vi "Populate Method Results.vi"(8 "error in (no error)":errorcluster, 10 "Test Method Result":refnum<class "Method Result.lvclass">, 11 "Test Tree In":refnum<class "Test Result Tree.lvclass">) -> (0 "error out":errorcluster, 2 "Test Method Result Out":refnum<class "Method Result.lvclass">, 3 "Test Tree Out":refnum<class "Test Result Tree.lvclass">)   [LabVIEW 2020, in "Test Result Tree.lvclass"]
uses:
  Test Result Tree/Test Result Tree.lvclass
  C:/Users/anton/Documents/GitHub/LUnit/source/Framework/Helper Classes/Test Tree/Test Tree.lvclass
  Result Classes/Method Result/Method Result.lvclass
  Test Tree.lvclass/Test Tree.ctl
  Result Classes/Method Result/Method Result.lvclass/Method Result.ctl
  Test Tree.lvclass
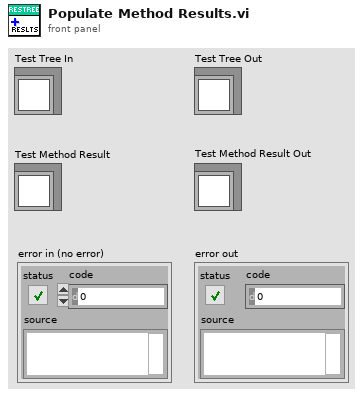
[diagram p1: front panel]
types:
  T1 = map{string, cluster{"Left Cell String":string, "Child Text":string[], "Item Indent":i32, "Child Only?":bool, "Glyph Index":i32}}
  T2 = typedef "Assertion Result.lvclass/Status.ctl" = enum16{"Pass", "Fail", "Error", "Skipped", "Setup Error", "Broken", "Teardown Error"}
  T3 = cluster{"Left Cell String":string, "Child Text":string[], "Item Indent":i32, "Child Only?":bool, "Glyph Index":i32}
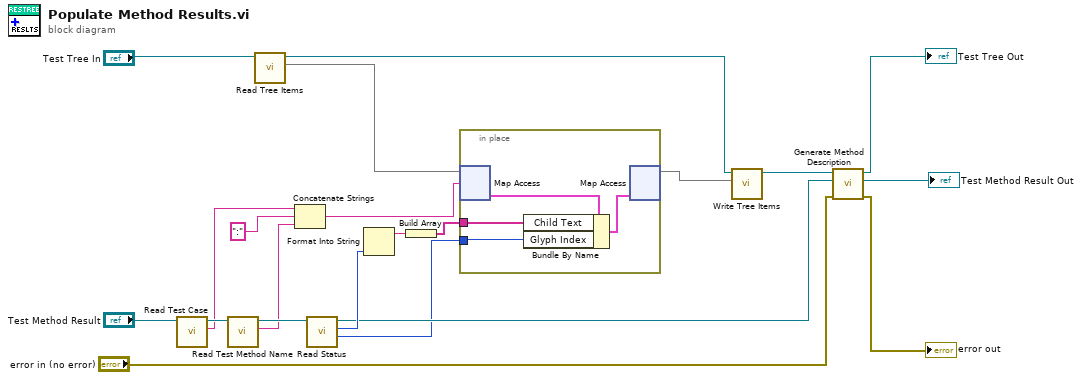
[diagram p0: block diagram]
diagram:
  n1 = call "Read Test Case.vi"("Method Result In"="Test Method Result") -> ("Test Case"=w18:string, "Method Result Out"=w19:refnum<class "Method Result.lvclass">)  [unwired: 9 in]
  n2 = call "Read Test Method Name.vi"("Method Result In"=w19) -> ("Test Method Name"=w14:string, "Method Result Out"=w21:refnum<class "Method Result.lvclass">)  [unwired: 9 in]
  n3 = call "Read Tree Items.vi"("Test Tree In"="Test Tree In") -> ("Tree Items"=w4:T1, "Test Tree Out"=w6:refnum<class "Test Result Tree.lvclass">)  [unwired: 9 in]
  n4 = Concatenate Strings(w18, ":" ("string"), w14) -> (w9:string)
  n5 = call "Read Status.vi"("Method Result In"=w21) -> ("Glyph Index"=w7:i32, "Status"=w16:T2, "Method Result Out"=w12:refnum<class "Method Result.lvclass">)  [unwired: 8 in]
  n6 = Format Into String(w16) -> (resulting string=w15:string)  [unwired: 3 in, 1 out]
  n7 = Build Array(w15) -> (w8:string[])
  n8 = in-place {
    in-place-border: w8 -> [w25]
    in-place-border: w7 -> [w24]
    n9 = in-place-map #1(w4, w9) -> (w23:T3)  [unwired: 1 in, 1 out]
    n10 = Bundle By Name(cluster=w23, "Child Text"=w25, "Glyph Index"=w24) -> (w22:T3)
    n11 = in-place-map #1(w22) -> (w3:T1)  [unwired: 1 in, 2 out]
  }
  n12 = call "Write Tree Items.vi"("Tree Items"=w3, "Test Tree In"=w6) -> ("Test Tree Out"=w2:refnum<class "Test Result Tree.lvclass">)  [unwired: 9 in]
  n13 = call "Generate Method Description.vi"("error in (no error)"="error in (no error)", "Test Method Result In"=w12, "Test Tree In"=w2) -> ("error out"=→"error out":errorcluster, "Test Method Result Out"=→"Test Method Result Out":refnum<class "Method Result.lvclass">, "Test Tree Out"=→"Test Tree Out":refnum<class "Test Result Tree.lvclass">)  [unwired: 6 in]
